vi "Send Update Load Forecast Longterm.vi"(7 "Message Priority (Normal)":T3=enum."Normal", 8 "error in (no error)":errorcluster, 10 "Load Power Forecast":T1, 11 "Message Enqueuer":refnum<class "Message Enqueuer.lvclass">) -> (0 "error out":errorcluster, 3 "Message Enqueuer out":refnum<class "Message Enqueuer.lvclass">)   [LabVIEW 2016, in "Optimization Framework.lvlib" / "Update Load Forecast Longterm Msg.lvclass"]
doc: "This VI sends the message to an actor."
uses:
  Update Load Forecast Longterm Msg.lvclass
  <vilib>/ActorFramework/Message Enqueuer/Message Enqueuer.lvclass
  <vilib>/ActorFramework/Message Enqueuer/Message Priority.ctl
  Optimization/Controls/Forecast Device Power.ctl
  Optimization/Controls/PDF Cluster.ctl
  C:/Program Files (x86)/National Instruments/LabVIEW 2016/vi.lib/ActorFramework/Message/Message.lvclass
  Update Load Forecast Longterm Msg.lvclass/Update Load Forecast Longterm Msg.ctl
  <vilib>/ActorFramework/Message Enqueuer/Message Enqueuer.lvclass/Message Enqueuer.ctl
  <vilib>/ActorFramework/Message Priority Queue/Priority Enqueue.vi
  Optimization/Optimization.lvclass
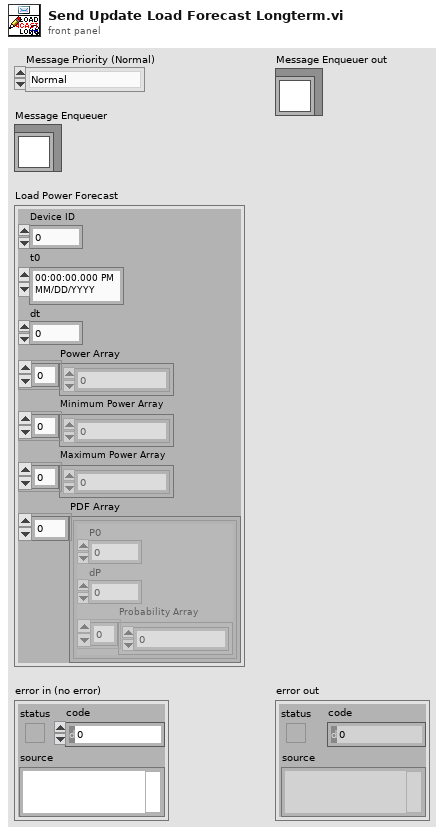
[diagram p1: front panel]
types:
  T1 = typedef "Optimization Framework.lvlib/Optimization.lvclass/Forecast Device Power.ctl" = cluster{"Device ID":u64, "t0":timestamp, "dt":dbl, "Power Array":dbl[], "Minimum Power Array":dbl[], "Maximum Power Array":dbl[], "PDF Array":T2[]}
  T2 = typedef "Optimization Framework.lvlib/Optimization.lvclass/PDF Cluster.ctl" = cluster{"P0":dbl, "dP":dbl, "Probability Array":dbl[]}
  T3 = typedef "Actor Framework.lvlib/Message Enqueuer.lvclass/Message Priority.ctl" = enum16{"Low", "Normal", "High"}
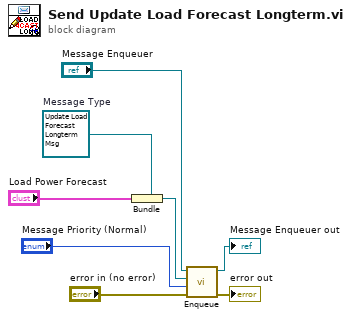
[diagram p0: block diagram]
diagram:
  w5 = refnum<class "Update Load Forecast Longterm Msg.lvclass"> refnum  # Message Type
  n1 = Bundle(cluster=w5, "Load Power Forecast") -> (w4:refnum<class "Update Load Forecast Longterm Msg.lvclass">)
  n2 = call <vilib>:"Enqueue.vi"("error in (no error)"="error in (no error)", "Message Priority (Normal)"="Message Priority (Normal)", "Message"=w4, "Message Enqueuer in"="Message Enqueuer") -> ("error out"=→"error out":errorcluster, "Message Enqueuer out"=→"Message Enqueuer out":refnum<class "Message Enqueuer.lvclass">)  [unwired: 6 in]
